vi "Database Update.vi"() -> ()   [LabVIEW 2012]
doc: "This example shows how you can update information in the FetchData table in a database named LabVIEW.mdb located in the LabVIEW examples>>database directory.\n\nThis VI is running when you open it. Select one of the names in the ring control and enter a new phone number. Press the Change button to complete the update and display the current data in the table."
uses:
  NI_Database_API_64.lvlib
  Connection.llb/DB Tools Open Connec (Path).vi
  _DB Variant To Data/Database Variant To Data.xnode
panel:
  out "Final Data":string[][](table)
  out "Initial Data":string[][](table)
  in  "change":bool
  in  "New phone number":string="555-1212"
  in  "Name":u16(ring) items=["Joe Smith", "Greg Myers", "Steve Jones", "Anne Harvey"]
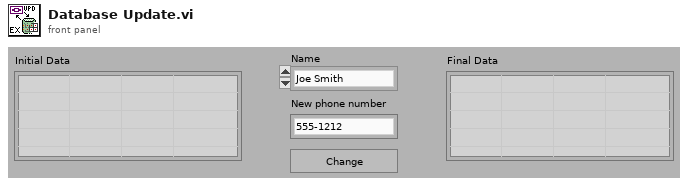
[diagram p1: front panel]
types:
  T1 = typedef "NI_Database_API_64.lvlib/Conn ObjectReference.ctl" = refnum<k1>
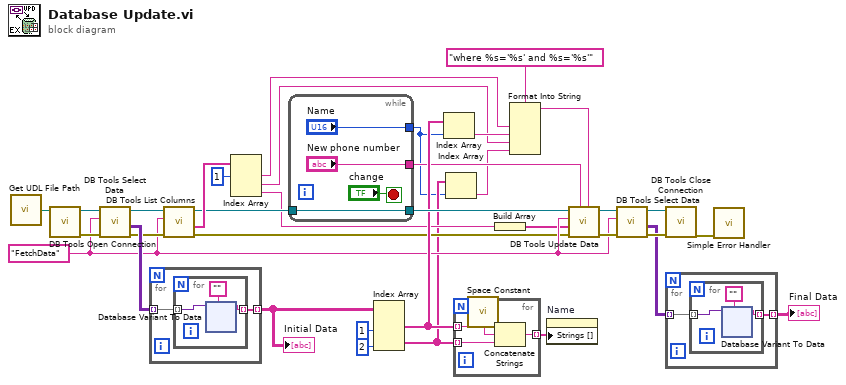
[diagram p0: block diagram]
diagram:
  w18 = "FetchData" ("table")
  n1 = call "Get UDL File Path.vi"() -> ("UDL file path"=w33:path)  [unwired: 1 in]
  n2 = call-poly "DB Tools Open Connection.vi"("connection information"=w33) -> ("error out"=w32:errorcluster, "connection reference"=w34:T1)  [unwired: 7 in]
  n3 = call "DB Tools Select Data.vi"("error in (no error)"=w32, "table"=w18, "connection reference"=w34) -> ("error out"=w19:errorcluster, "data"=w35:variant[][], "connection reference out"=w20:T1)  [unwired: 3 in]
  n4 = for {
    tunnel: w35 -> [w37] mode=indexing
    tunnel: [w36] -> w12 mode=indexing
    n5 = for {
      tunnel: w37 -> [w39] mode=indexing
      tunnel: [w38] -> w36 mode=indexing
      n6 = xnode "Database Variant To Data"("database variant"=w39, "type"="") -> ("data"=w38:string)  [unwired: 1 in, 1 out]
    }
  }
  "Initial Data" <- w12
  n7 = call "DB Tools List Columns.vi"("error in (no error)"=w19, "table"=w18, "connection reference"=w20) -> ("error out"=w15:errorcluster, "columns"=w16:string[], "connection reference out"=w14:T1)  [unwired: 1 in, 1 out]
  n8 = Index Array(array=w16, index #1=1 ("disabled index (col)")) -> (element #1=w5:string, element #2=w3:string, element #3=w9:string)  [unwired: 2 in]
  n9 = while {
    tunnel: w14 -> [w76]
    tunnel: [w76] -> w22
    tunnel: ["Name"] -> w7
    tunnel: ["New phone number"] -> w10
    stop <- "change" stop-if-true
  }
  n10 = Index Array(array=w12, index (col) #1=1 ("disabled index (col)"), index (col) #2=2 ("index (col)")) -> (element #1=w21:string[], element #2=w8:string[])  [unwired: 2 in]
  n11 = Index Array(array=w21, index=w7) -> (element=w4:string)
  n12 = Index Array(array=w8, index=w7) -> (element=w2:string)
  n13 = for {
    tunnel: w21 -> [w79] mode=indexing
    tunnel: w8 -> [w78] mode=indexing
    tunnel: [w77] -> w29 mode=indexing
    n14 = call <vilib>:"Space Constant.vi"() -> ("String"=w80:string)
    n15 = Concatenate Strings(w79, w80, w78) -> (w77:string)
  }
  n16 = Build Array(w9) -> (w13:string[])
  n17 = Format Into String(format string="where %s='%s' and %s='%s'", w5, w4, w3, w2) -> (resulting string=w1:string)  [unwired: 2 in, 1 out]
  n18 = property on="Name" class="Ring (strict)"("Strings []"=w29) -> ()  [unwired: 2 in, 2 out]
  n19 = call "DB Tools Update Data.vi"("condition"=w1, "data"=w10, "error in (no error)"=w15, "columns"=w13, "table"=w18, "connection reference"=w22) -> ("error out"=w27:errorcluster, "connection reference out"=w28:T1)  [unwired: 4 in]
  n20 = call "DB Tools Select Data.vi"("error in (no error)"=w27, "table"=w18, "connection reference"=w28) -> ("error out"=w25:errorcluster, "data"=w24:variant[][], "connection reference out"=w26:T1)  [unwired: 3 in]
  n21 = call "DB Tools Close Connection.vi"("error in (no error)"=w25, "connection reference"=w26) -> ("error out"=w23:errorcluster)  [unwired: 5 in]
  n22 = for {
    tunnel: w24 -> [w82] mode=indexing
    tunnel: [w81] -> w11 mode=indexing
    n23 = for {
      tunnel: w82 -> [w84] mode=indexing
      tunnel: [w83] -> w81 mode=indexing
      n24 = xnode "Database Variant To Data"("database variant"=w84, "type"="") -> ("data"=w83:string)  [unwired: 1 in, 1 out]
    }
  }
  "Final Data" <- w11
  n25 = call <vilib>:"Simple Error Handler.vi"("error in (no error)"=w23) -> ()  [unwired: 4 in, 5 out]
